vi "TimerPause.vi"(8 "Error In":errorcluster, 10 "Time Target (s)":dbl=4.0, 11 "Timer Mode":T1) -> (0 "Error Out":errorcluster, 2 "Has Time Elapsed":bool, 3 "Elapsed Time (s.ss)":dbl)   [LabVIEW 2019]
doc: "CLD 3 Exercise"
uses:
  Controls/TimerModes.ctl
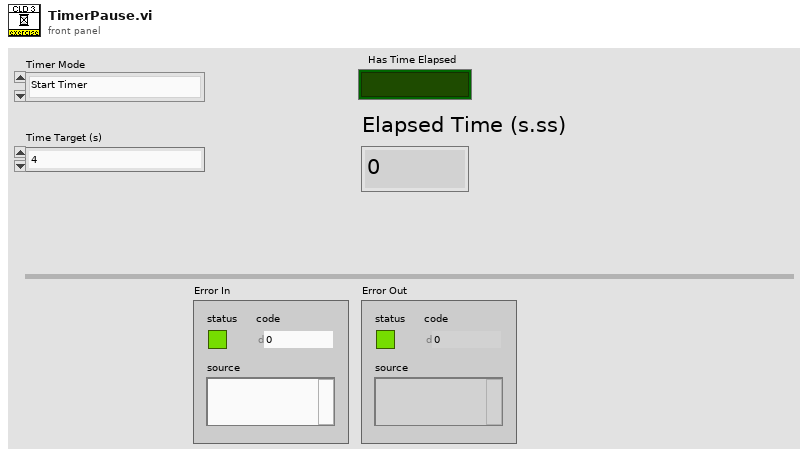
[diagram p1: front panel]
types:
  T1 = typedef "TimerModes.ctl" = enum16{"Start Timer", "Read Time", "Pause", "Resume"}
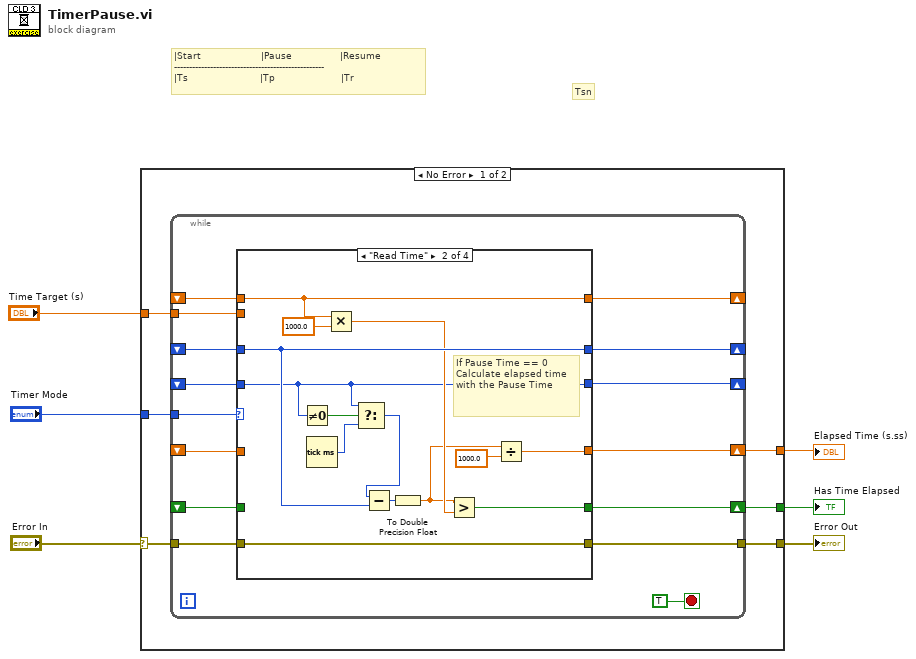
[diagram p0: block diagram]
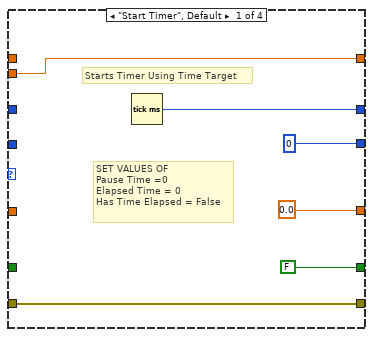
[diagram p2: hidden frame]
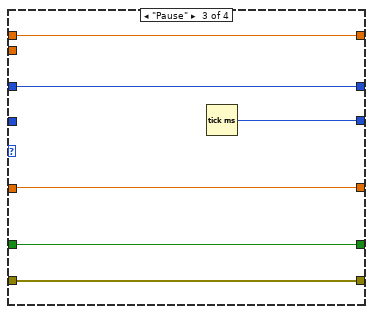
[diagram p3: hidden frame]
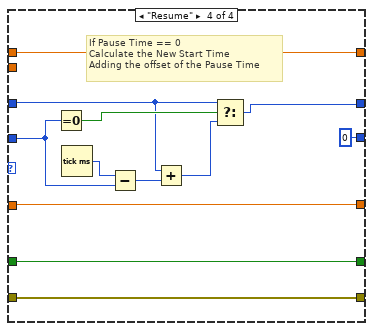
[diagram p4: hidden frame]
diagram:
  # "Tsn"
  # "|Start                    |Pause                |Resume\n--------------------------------------------------\n|Ts                        |Tp                      |Tr"
  n1 = case shown="No Error" "Error In" {
    selector: "Error In" -> [w12 w66]
    tunnel: [w11 w66] -> w5
    tunnel: "Timer Mode" -> [w10 _]
    tunnel: "Time Target (s)" -> [w9 _]
    tunnel: [w8 _] -> w2
    tunnel: [w7 _] -> w1
    frame No Error {
      n2 = while {
        tunnel: w12 -> [w27]
        tunnel: [w26] -> w11
        tunnel: w10 -> [w25]
        shift-right: [w23] -> _
        shift-left: _ -> [w22]
        shift-right: [w21] -> _
        shift-left: _ -> [w24]
        tunnel: w9 -> [w20]
        shift-right: [w18] -> w7
        shift-left: _ -> [w17]
        shift-right: [w15] -> _
        shift-left: _ -> [w14]
        shift-right: [w19] -> w8
        shift-left: _ -> [w13]
        stop <- TRUE stop-if-true
        n3 = case shown="\"Read Time\"" w25 {
          tunnel: [w33 w47 w53 w65] -> w26
          tunnel: w27 -> [w33 w47 w53 w65]
          tunnel: w24 -> [_ w44 w52 w64]
          tunnel: [w32 w44 w52 w64] -> w21
          tunnel: [w30 w46 w50 w54] -> w23
          tunnel: w22 -> [_ w46 w50 w56]
          tunnel: w20 -> [w32 _ _ _]
          tunnel: [FALSE w41 w48 w60] -> w19
          tunnel: [0.0 w40 w51 w63] -> w18
          tunnel: w17 -> [_ _ w51 w63]
          tunnel: [u32 0 ("millisecond timer value") w36 w49 u32 0 ("millisecond timer value")] -> w15
          tunnel: w14 -> [_ w36 _ w59]
          tunnel: w13 -> [_ _ w48 w60]
          frame "Start Timer", Default {
            # "SET VALUES OF\nPause Time =0\nElapsed Time = 0\nHas Time Elapsed = False"
            # "Starts Timer Using Time Target"
            n4 = Tick Count (ms)() -> (millisecond timer value=w30:u32)
          }
          frame "Read Time" {
            # "If Pause Time == 0\nCalculate elapsed time \nwith the Pause Time"
            n5 = Not Equal To 0?(x=w36) -> (x != 0?=w37:bool)
            n6 = Tick Count (ms)() -> (millisecond timer value=w35:u32)
            n7 = Multiply(x=w44, y=1000.0) -> (x*y=w42:dbl)
            n8 = Select(t=w36, s=w37, f=w35) -> (s? t:f=w34:u32)
            n9 = Subtract(x=w34, y=w46) -> (x-y=w45:u32)
            n10 = To Double Precision Float(number=w45) -> (double precision float=w39:dbl)
            n11 = Greater?(x=w39, y=w42) -> (0:w41:bool)
            n12 = Divide(x=w39, y=1000.0) -> (x/y=w40:dbl)
          }
          frame "Pause" {
            n13 = Tick Count (ms)() -> (millisecond timer value=w49:u32)
          }
          frame "Resume" {
            # "If Pause Time == 0\nCalculate the New Start Time \nAdding the offset of the Pause Time"
            n14 = Equal To 0?(x=w59) -> (x = 0?=w58:bool)
            n15 = Tick Count (ms)() -> (millisecond timer value=w57:u32)
            n16 = Subtract(x=w57, y=w59) -> (x-y=w62:u32)
            n17 = Add(x=w56, y=w62) -> (x+y=w55:u32)
            n18 = Select(t=w56, s=w58, f=w55) -> (s? t:f=w54:u32)
          }
        }
      }
    }
    frame Error {
    }
  }
  "Error Out" <- w5
  "Has Time Elapsed" <- w2
  "Elapsed Time (s.ss)" <- w1
